vi "Get Contour Color.vi"(5 "Opacity":sgl, 7 "Contour Property In":T1={"Contour Type"=enum."Contour with surface", "Axis Basis"=enum."X-Axis", "Level List"=[], "Level Mode"=enum."Levels", "Levels"=0, "Interval"=0.0}, 8 "Line Color":u32(colorbox), 9 "Actual Range":T3, 10 "Color Ramp Cluster":T4={"Color Ramp Style"=enum."None", "Color Ramp Array"=[16711934, 393471, 57855, 4390754, 16449346, 16744722, 16711680], "Color Ramp Index"=[45, 91, 133, 175, 219, 255], "Interpolate?"=FALSE, "Logarithm?"=FALSE}, 11 "Contour Vertex Array":cluster{"X":sgl, "Y":sgl, "Z":sgl}[](array[cluster])) -> (1 "Color Binding Mode":T2(ring)=enum."Per Primitive", 3 "Color Array Out":cluster{"R":sgl, "G":sgl, "B":sgl, "A":sgl}[](array[cluster]))   [LabVIEW 2017, in "3D Contour.lvclass"]
uses:
  <vilib>/Math Plots/3D Math Plots/3D Contour/3D Contour/3D Contour.lvclass
  <vilib>/Math Plots/3D Math Plots/3D Plot/3D Plot/Typedef/Color Ramp Cluster.ctl
  <vilib>/Math Plots/3D Math Plots/3D Plot/3D Plot/Typedef/Range Clusters.ctl
  <vilib>/Math Plots/3D Math Plots/3D Plot/3D Plot/3D Plot.lvclass
  <vilib>/picture/3D Picture Control/NI_3D Picture Control.lvlib
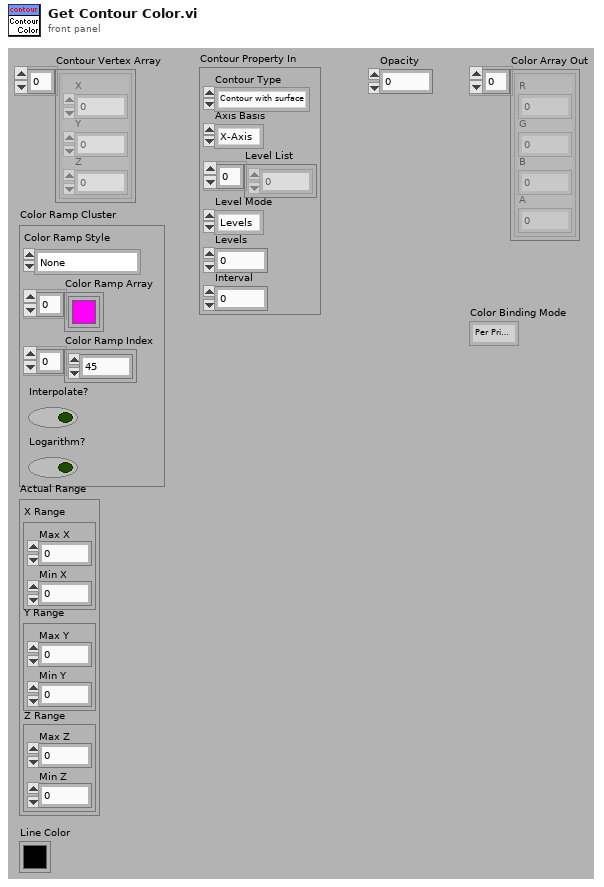
[diagram p1: front panel]
types:
  T1 = cluster{"Contour Type":enum16{"Contour", "Contour with surface"}, "Axis Basis":enum16{"X-Axis", "Y-Axis", "Z-Axis"}, "Level List":sgl[], "Level Mode":enum16{"Levels", "Interval", "Level List"}, "Levels":u16, "Interval":sgl}
  T2 = enum16{"Overall", "Per Primitive", "Per Vertex", "Binding Off"}
  T3 = typedef "3D Plot.lvclass/Range Clusters.ctl" = cluster{"X Range":cluster{"Max X":sgl, "Min X":sgl}, "Y Range":cluster{"Max Y":sgl, "Min Y":sgl}, "Z Range":cluster{"Max Z":sgl, "Min Z":sgl}}
  T4 = typedef "3D Plot.lvclass/Color Ramp Cluster.ctl" = cluster{"Color Ramp Style":enum16{"None", "Shaded", "Color spectrum", "Grey scale", "Custom"}, "Color Ramp Array":u32[], "Color Ramp Index":i32[], "Interpolate?":bool, "Logarithm?":bool}
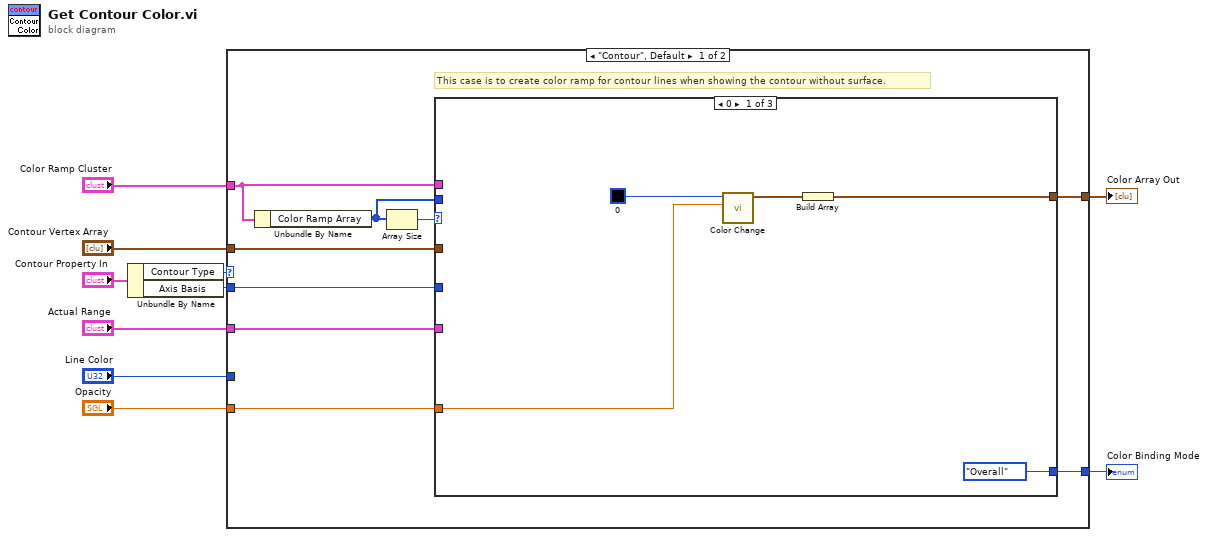
[diagram p0: block diagram]
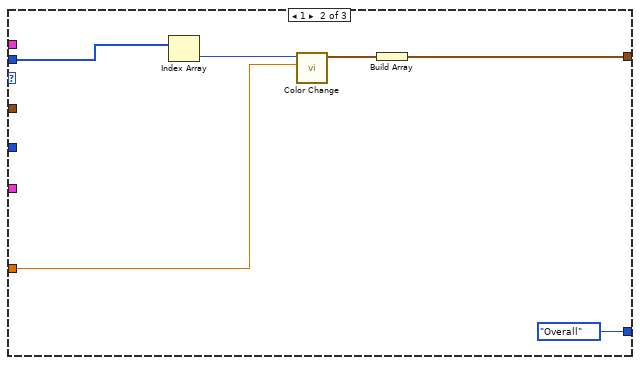
[diagram p2: hidden frame]
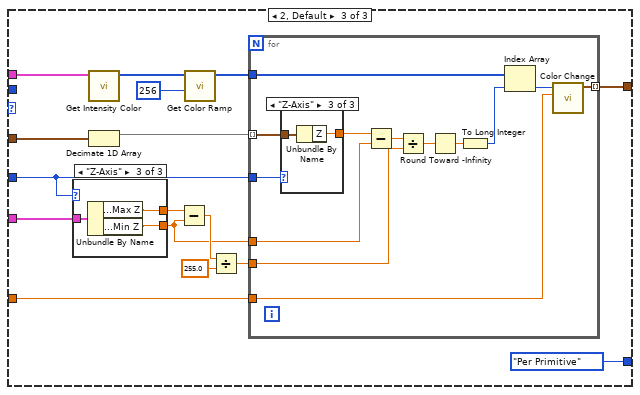
[diagram p3: hidden frame]
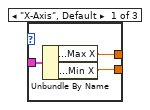
[diagram p4: hidden frame]
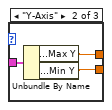
[diagram p5: hidden frame]
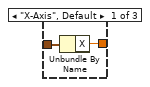
[diagram p6: hidden frame]
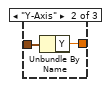
[diagram p7: hidden frame]
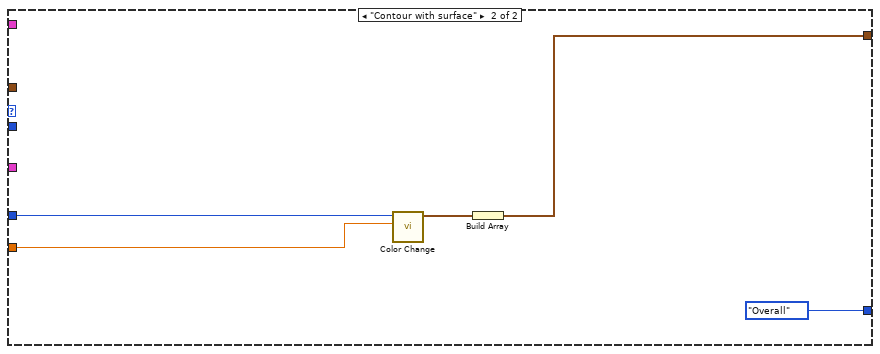
[diagram p8: hidden frame]
diagram:
  n1 = Unbundle By Name("Contour Property In") -> ("Contour Type"=w2:enum16{"Contour", "Contour with surface"}, "Axis Basis"=w3:enum16{"X-Axis", "Y-Axis", "Z-Axis"})
  n2 = case shown="\"Contour\", Default" w2 {
    tunnel: "Contour Vertex Array" -> [w19 _]
    tunnel: "Opacity" -> [w18 w78]
    tunnel: [w17 w76] -> w8
    tunnel: "Color Ramp Cluster" -> [w11 _]
    tunnel: "Actual Range" -> [w16 _]
    tunnel: [w15 T2."Overall" ("Color Binding Mode")] -> w5
    tunnel: w3 -> [w14 _]
    tunnel: "Line Color" -> [_ w79]
    frame "Contour", Default {
      # "This case is to create color ramp for contour lines when showing the contour without surface."
      n3 = Unbundle By Name(w11) -> ("Color Ramp Array"=w13:u32[])
      n4 = Array Size(array=w13) -> (size(s)=w12:i32)
      n5 = case shown="0" w12 {
        tunnel: w19 -> [_ _ w46]
        tunnel: w18 -> [w22 w27 w44]
        tunnel: [w21 w26 w43] -> w17
        tunnel: w16 -> [_ _ w40]
        tunnel: [T2."Overall" ("Color Binding Mode") T2."Overall" ("Color Binding Mode") T2."Per Primitive" ("Color Binding Mode")] -> w15
        tunnel: w14 -> [_ _ w32]
        tunnel: w13 -> [_ w28 _]
        tunnel: w11 -> [_ _ w31]
        frame 0 {
          n6 = call <vilib>:"Color Change.vi"("Alpha"=w22, "Color"=u32 0) -> ("RGBA"=w24:cluster{"R":sgl, "G":sgl, "B":sgl, "A":sgl})  [unwired: 9 out]
          n7 = Build Array(w24) -> (w21:cluster{"R":sgl, "G":sgl, "B":sgl, "A":sgl}[])
        }
        frame 1 {
          n8 = Index Array(array=w28) -> (element=w30:u32)  [unwired: 1 in]
          n9 = call <vilib>:"Color Change.vi"("Alpha"=w27, "Color"=w30) -> ("RGBA"=w29:cluster{"R":sgl, "G":sgl, "B":sgl, "A":sgl})  [unwired: 9 out]
          n10 = Build Array(w29) -> (w26:cluster{"R":sgl, "G":sgl, "B":sgl, "A":sgl}[])
        }
        frame 2, Default {
          n11 = case shown="\"Z-Axis\"" w32 {
            tunnel: w40 -> [w49 w52 w55]
            tunnel: [w48 w51 w54] -> w37
            tunnel: [w47 w50 w53] -> w36
            frame "X-Axis", Default {
              n12 = Unbundle By Name(w49) -> ("X Range.Max X"=w48:sgl, "X Range.Min X"=w47:sgl)
            }
            frame "Y-Axis" {
              n13 = Unbundle By Name(w52) -> ("Y Range.Max Y"=w51:sgl, "Y Range.Min Y"=w50:sgl)
            }
            frame "Z-Axis" {
              n14 = Unbundle By Name(w55) -> ("Z Range.Max Z"=w54:sgl, "Z Range.Min Z"=w53:sgl)
            }
          }
          n15 = call <vilib>:"Get Intensity Color.vi"("Color Ramp Cluster"=w31) -> ("Intensity Color"=w42:u32[])  [unwired: 3 in, 7 out]
          n16 = Decimate 1D Array(w46) -> (w41:cluster{"X":sgl, "Y":sgl, "Z":sgl}[])  [unwired: 1 out]
          n17 = Subtract(x=w37, y=w36) -> (x-y=w39:sgl)
          n18 = call <vilib>:"Get Color Ramp.vi"("Number of Colors"=256, "Color Ramp Array"=w42) -> ("RGB Array"=w45:u32[])  [unwired: 1 in, 8 out]
          n19 = Divide(x=w39, y=sgl 255.0) -> (x/y=w35:sgl)
          n20 = for {
            tunnel: w45 -> [w68]
            tunnel: w44 -> [w66]
            tunnel: [w65] -> w43 mode=indexing
            tunnel: w41 -> [w61] mode=indexing
            tunnel: w36 -> [w58]
            tunnel: w35 -> [w57]
            tunnel: w32 -> [w60]
            n21 = case shown="\"Z-Axis\"" w60 {
              tunnel: w61 -> [w70 w72 w74]
              tunnel: [w69 w71 w73] -> w59
              frame "X-Axis", Default {
                n22 = Unbundle By Name(w70) -> ("X"=w69:sgl)
              }
              frame "Y-Axis" {
                n23 = Unbundle By Name(w72) -> ("Y"=w71:sgl)
              }
              frame "Z-Axis" {
                n24 = Unbundle By Name(w74) -> ("Z"=w73:sgl)
              }
            }
            n25 = Subtract(x=w59, y=w58) -> (x-y=w62:sgl)
            n26 = Divide(x=w62, y=w57) -> (x/y=w64:sgl)
            n27 = Round Toward -Infinity(1:w64) -> (0:w63:sgl)
            n28 = To Long Integer(number=w63) -> (32bit integer=w56:i32)
            n29 = Index Array(array=w68, index=w56) -> (element=w67:u32)
            n30 = call <vilib>:"Color Change.vi"("Alpha"=w66, "Color"=w67) -> ("RGBA"=w65:cluster{"R":sgl, "G":sgl, "B":sgl, "A":sgl})  [unwired: 9 out]
          }
        }
      }
    }
    frame "Contour with surface" {
      n31 = call <vilib>:"Color Change.vi"("Alpha"=w78, "Color"=w79) -> ("RGBA"=w77:cluster{"R":sgl, "G":sgl, "B":sgl, "A":sgl})  [unwired: 9 out]
      n32 = Build Array(w77) -> (w76:cluster{"R":sgl, "G":sgl, "B":sgl, "A":sgl}[])
    }
  }
  "Color Array Out" <- w8
  "Color Binding Mode" <- w5
